vi "Launch Hardware Settings.vi"(8 "error in (no error)":errorcluster, 10 "Device":i32, 11 "Measurement UI in":refnum<class "Measurement UI.lvclass">) -> (0 "error out":errorcluster, 3 "Measurement UI out":refnum<class "Measurement UI.lvclass">)   [LabVIEW 2016, in "Measurement UI.lvlib" / "Measurement UI.lvclass"]
uses:
  Measurement UI.lvclass
  C:/Program Files (x86)/National Instruments/LabVIEW 2016/vi.lib/ActorFramework/Actor/Actor.lvclass
  Measurement UI.lvclass/Measurement UI.ctl
  <vilib>/ActorFramework/Actor/Actor.lvclass/Actor.ctl
  Controller Messages/Launch Hardware Settings Dialog Msg/Launch Hardware Settings Dialog Msg.lvclass/Launch Hardware Settings Dialog Msg.ctl
  <vilib>/ActorFramework/Message Enqueuer/Message Enqueuer.lvclass/Message Enqueuer.ctl
  Read Multimeter.vi
  Accessors/Read Digitizer.vi
  Accessors/Read Function Generator.vi
  Accessors/Read Power Supply.vi
  Accessors/Read Measurement.vi
  <vilib>/ActorFramework/Message Enqueuer/Enqueue.vi
  Controller Messages/Launch Hardware Settings Dialog Msg/Launch Hardware Settings Dialog Msg.lvclass
  C:/Program Files (x86)/National Instruments/LabVIEW 2016/vi.lib/ActorFramework/Message/Message.lvclass
  <vilib>/ActorFramework/Message Priority Queue/Priority Enqueue.vi
  <vilib>/ActorFramework/Actor/Actor.lvclass
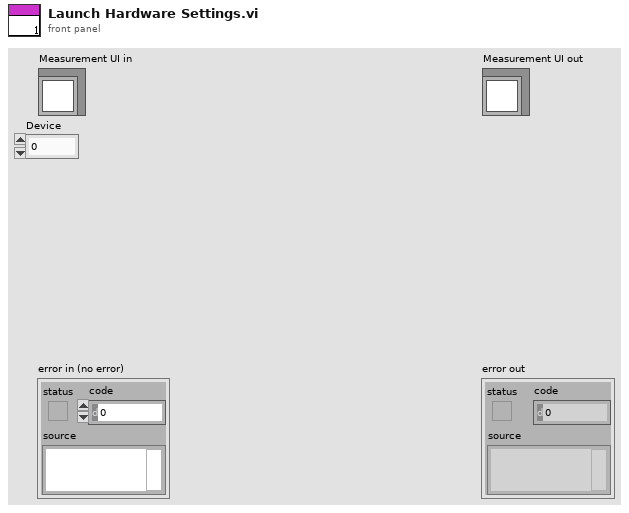
[diagram p1: front panel]
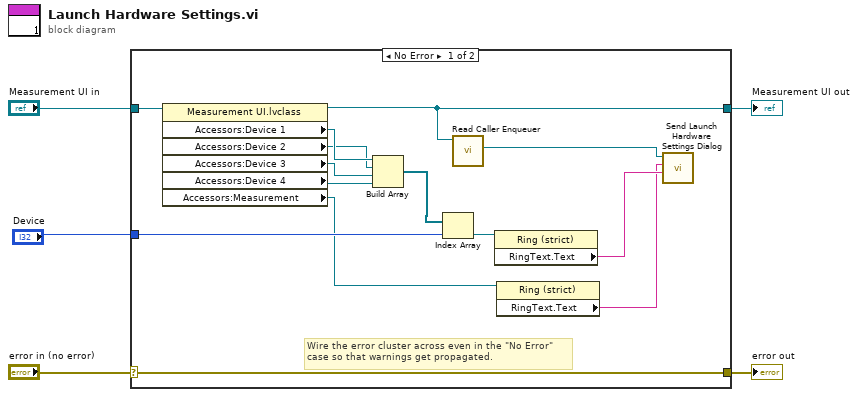
[diagram p0: block diagram]
diagram:
  n1 = case shown="No Error" "error in (no error)" {
    selector: "error in (no error)" -> [w19 w21]
    tunnel: [w19 w21] -> w4
    tunnel: [w17 w20] -> w2
    tunnel: "Measurement UI in" -> [w18 w20]
    tunnel: "Device" -> [w11 _]
    frame No Error {
      # "Wire the error cluster across even in the \"No Error\"\ncase so that warnings get propagated."
      n2 = property class="Measurement UI.lvclass"(reference=w18) -> (reference out=w17:refnum<class "Measurement UI.lvclass">, "Accessors:Device 1"=w16:refnum<vi>, "Accessors:Device 2"=w15:refnum<vi>, "Accessors:Device 3"=w14:refnum<vi>, "Accessors:Device 4"=w13:refnum<vi>, "Accessors:Measurement"=w9:refnum<vi>)  [unwired: 1 in, 1 out]
      n3 = Build Array(w16, w15, w14, w13) -> (w12:refnum<vi>[])
      n4 = Index Array(array=w12, index=w11) -> (element=w10:refnum<vi>)
      n5 = call <vilib>:"Read Caller Enqueuer.vi"("Actor"=w17) -> ("Caller Enqueuer"=w6:refnum<class "Message Enqueuer.lvclass">)  [unwired: 10 in]
      n6 = property class="Ring (strict)"(reference=w10) -> ("RingText.Text"=w8:string)  [unwired: 1 in, 2 out]
      n7 = property class="Ring (strict)"(reference=w9) -> ("RingText.Text"=w7:string)  [unwired: 1 in, 2 out]
      n8 = call "Send Launch Hardware Settings Dialog.vi"("Device"=w8, "Msmt"=w7, "Message Enqueuer"=w6) -> ()  [unwired: 7 in, 2 out]
    }
    frame Error {
    }
  }
  "error out" <- w4
  "Measurement UI out" <- w2
